vi "nufern test 1.vi"() -> ()   [LabVIEW 2016]
uses:
  <vilib>/Instr/_visa.llb/VISA Configure Serial Port (Instr).vi
panel:
  out "string to crc":string
  out "CRC2":i32 format="0x%x"
  out "concatenated string":string
  in  "PAPA Address":i8=10 format="0x%02x"
  in  "Calibration":u16(ring)=128 format="0x%x" items=["Set Photodiode Threshold"=128, "Get All Photodiode Thresholds"=129, "Set Photodiode Trimpot Setpoint"=130, "Get All Photodiode Trimpot Setpoints"=131, "Set Preamp Pump Current Setpoint"=132, "Get All Preamp Pump Current Setpoints"=133, "Set Temperature Sensor Warning Threshold"=134, "Get Temperature Sensor Warning Threshold"=135, "Set Temperature Sensor Fault Threshold"=136, "Get Temperature Sensor Fault Threshold"=137, "Set HPE Photodiode Auto Threshold Delay"=138, "Get HPE Photodiode Auto Threshold Delay"=139]
  in  "Extended Operation":u16(ring)=67 format="0x%x" items=["Set HPE Photodiode Signal Drop Tolerance"=67, "Get HPE Photodiode Signal Drop Tolerance"=68, "Switch HPE Photodiode Fault Enable"=69, "Get Temperature Sensor Status"=70, "Switch Communication Timeout Enable"=71]
  in  "Logistics":u16(ring)=65 format="0x%x" items=["Set RS-485 Address"=65, "Get RS-485 Address"=66]
  in  "Common Operation":u16(ring)=4 format="0x%d" items=["Undefined", "Query: Get Unit Information", "Cmd: Emission On", "Cmd: Emission Off", "Query: Get Basic Status", "Query: Get Core Status", "Query: Get Extended Status", "Cmd: Clear Faults", "Cmd: Set Power Mode"]
  out "error out":errorcluster
  in  "error in (no error)":errorcluster
  in  "baud rate (9600)":u32=115200
  in  "VISA resource name":refnum<visa-resource-name>
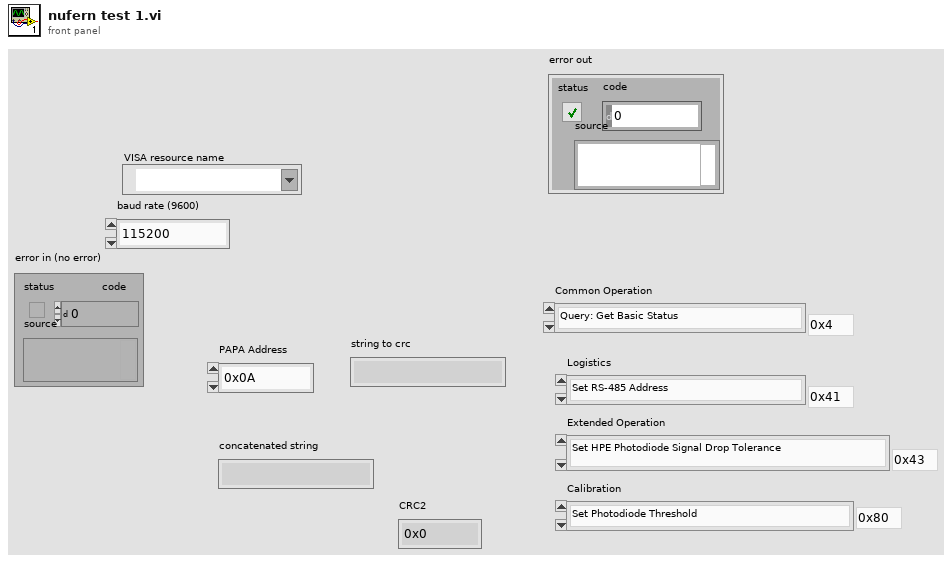
[diagram p1: front panel]
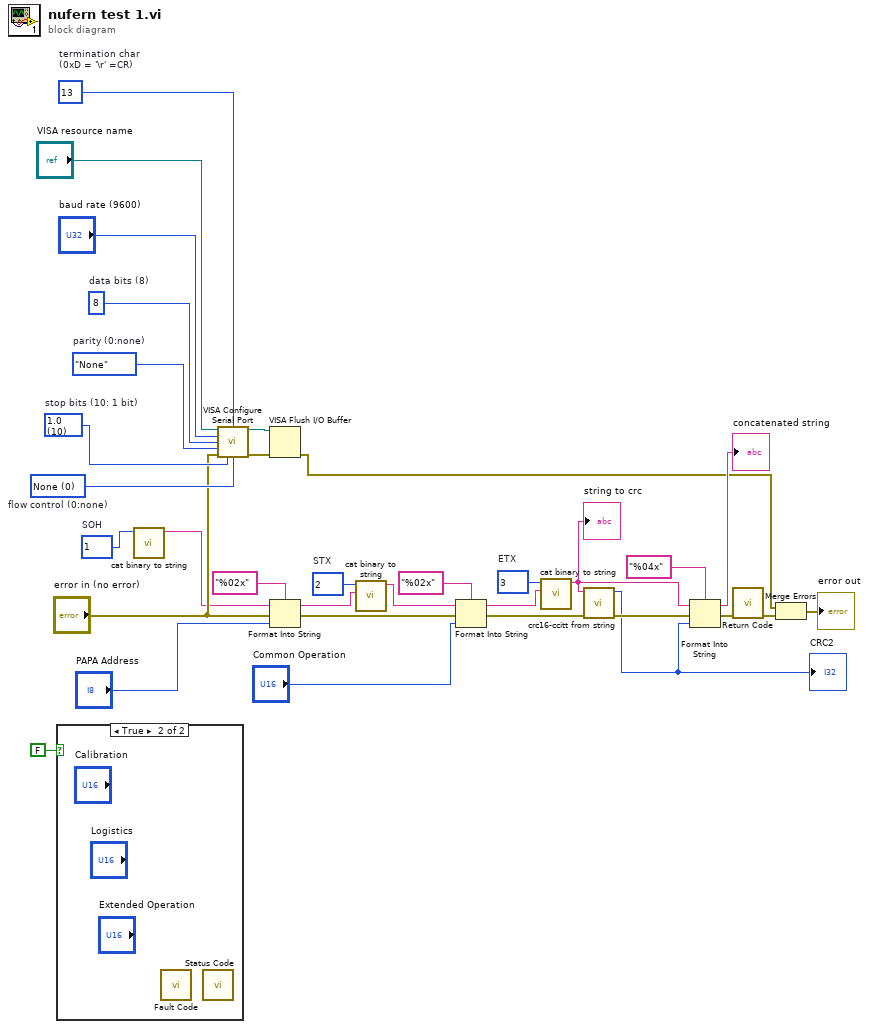
[diagram p0: block diagram]
diagram:
  w24 = u8 13  # termination char (0xD = '\r' =CR)
  w12 = 3  # ETX
  w4 = 2  # STX
  w2 = 1  # SOH
  w28 = u16 0 items=["None", "XON/XOFF", "RTS/CTS", "XON/XOFF & RTS/CTS", "DTR/DSR", "XON/XOFF & DTR/DSR"]  # flow control (0:none)
  w29 = u16 10 items=["1.0"=10, "1.5"=15, "2.0"=20]  # stop bits (10: 1 bit)
  w30 = enum16{"None", "Odd", "Even", "Mark", "Space"}."None"  # parity (0:none)
  w31 = u16 8  # data bits (8)
  n1 = case shown="True" FALSE ("Boolean") {
    frame False {
    }
    frame True {
      n2 = call "Fault Code.vi"() -> ()  [unwired: 10 in, 2 out]
      n3 = call "Status Code.vi"() -> ()  [unwired: 10 in, 2 out]
    }
  }
  n4 = call "cat binary to string.vi"("ETX"=w2) -> ("String out"=w1:string)  [unwired: 10 in]
  n5 = call-poly "VISA Configure Serial Port"("VISA resource name"="VISA resource name", "termination char\n(0xA = '\\n' = LF)"=w24, "baud rate (9600)"="baud rate (9600)", "data bits (8)"=w31, "parity (0:none)"=w30, "error in (no error)"="error in (no error)", "stop bits (10: 1 bit)"=w29, "flow control (0:none)"=w28) -> ("VISA resource name out"=w26:refnum<visa-resource-name>, "error out"=w27:errorcluster)  [unwired: 6 in]
  n6 = VISA Flush I/O Buffer(VISA resource name=w26, error in (no error)=w27) -> (error out=w15:errorcluster)  [unwired: 1 in, 1 out]
  n7 = Format Into String(format string="%02x", initial string=w1, error in="error in (no error)", "PAPA Address") -> (resulting string=w5:string, error out=w7:errorcluster)
  n8 = call "cat binary to string.vi"("String in"=w5, "ETX"=w4) -> ("String out"=w3:string)  [unwired: 9 in]
  n9 = Format Into String(format string="%02x", initial string=w3, error in=w7, "Common Operation") -> (resulting string=w13:string, error out=w10:errorcluster)
  n10 = call "cat binary to string.vi"("String in"=w13, "ETX"=w12) -> ("String out"=w11:string)  [unwired: 9 in]
  "string to crc" <- w11
  n11 = call "crc16-ccitt from string.vi"("error in (no error)"=w10, "String"=w11) -> ("error out"=w9:errorcluster, "CRC Out"=w8:i32)  [unwired: 8 in]
  "CRC2" <- w8
  n12 = Format Into String(format string="%04x", initial string=w11, error in=w9, w8) -> (resulting string=→"concatenated string":string, error out=w14:errorcluster)
  n13 = call "Return Code.vi"("error in (no error)"=w14) -> ("error out"=w25:errorcluster)  [unwired: 9 in, 1 out]
  n14 = Merge Errors(w15, w25) -> (→"error out":errorcluster)
